vi "DetectDaxsonics.vi"(11 "Main Digitizer":T1=enum."NI Digitizer") -> (1 "Trig Slope":u16(ring) items=["Positive", "Negative"], 2 "Offset Delay (us)":dbl)   [LabVIEW 2022 SP3]
uses:
  Digitizers/-DigitizerRoutines/Digitizer.ctl
  Daxsonics_Pulsers.ctl
  PulserGlobals.vi
panel:
  out "Daxsonics Present":refnum<visa-resource-name>[](array[refnum])
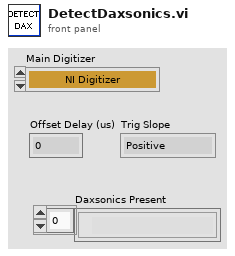
[diagram p1: front panel]
types:
  T1 = typedef "Digitizer.ctl" = enum16{"Acqiris Digitizer", "NI Digitizer", "LeCroy", "GaGe", "AlazarTech", "No Digitizer", "Teledyne"}
  T2 = typedef "Daxsonics_Pulsers.ctl" = enum16{"BP1", "BP2_A", "BP2_B", "10ERS8", "New2021"}
  T3 = enum16{"Left Button", "Center Button", "Right Button", "Window Close"}
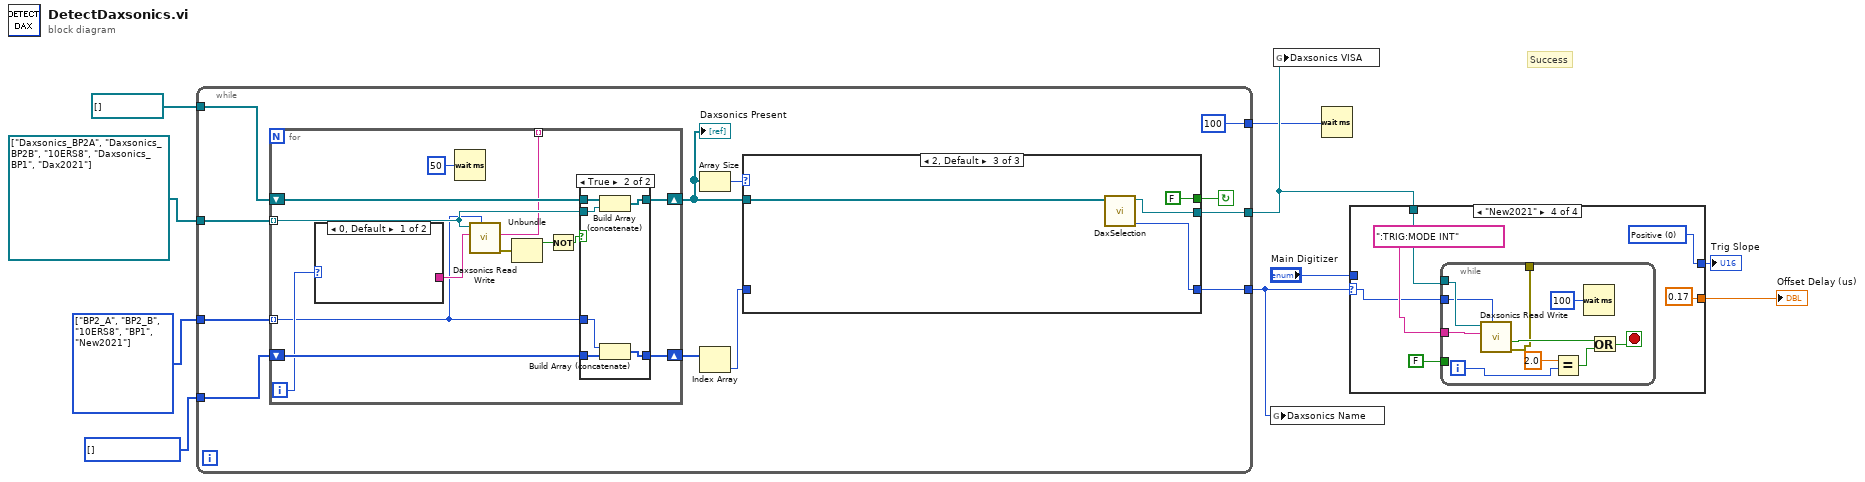
[diagram p0: block diagram]
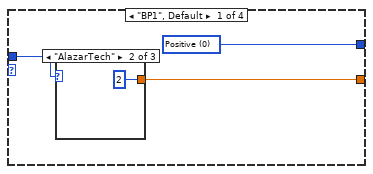
[diagram p2: hidden frame]
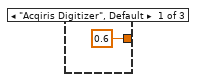
[diagram p3: hidden frame]
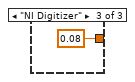
[diagram p4: hidden frame]
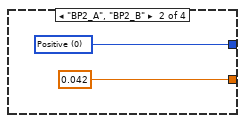
[diagram p5: hidden frame]
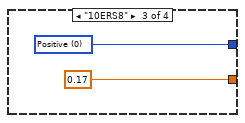
[diagram p6: hidden frame]
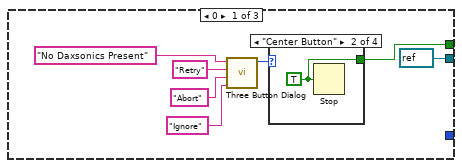
[diagram p7: hidden frame]
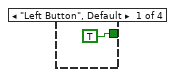
[diagram p8: hidden frame]
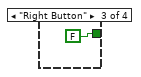
[diagram p9: hidden frame]
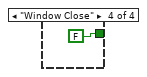
[diagram p10: hidden frame]
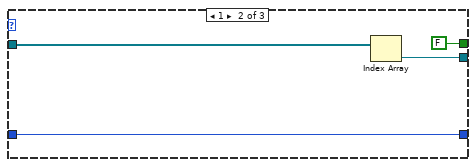
[diagram p11: hidden frame]
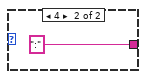
[diagram p12: hidden frame]
diagram:
  w4 = T2[] [] items=["BP1", "BP2_A", "BP2_B", "10ERS8", "New2021"]
  w5 = T2[] [enum."BP2_A", enum."BP2_B", enum."10ERS8", enum."BP1", enum."New2021"] items=["BP1", "BP2_A", "BP2_B", "10ERS8", "New2021"]
  # "Success"
  n1 = while {
    tunnel: [w20] -> w2
    tunnel: [w19] -> w7
    tunnel: refnum<visa-resource-name>[] ["Daxsonics_BP2A", "Daxsonics_BP2B", "10ERS8", "Daxsonics_BP1", "Dax2021"] -> [w15]
    tunnel: w5 -> [w14]
    tunnel: w4 -> [w13]
    tunnel: refnum<visa-resource-name>[] [] -> [w12]
    tunnel: [u32 100 ("milliseconds to wait")] -> w1
    stop <- w16 continue-if-true
    n2 = for {
      tunnel: w15 -> [w50] mode=indexing
      shift-right: [w51] -> w21
      shift-left: w12 -> [w53]
      tunnel: w14 -> [w42] mode=indexing
      shift-right: [w47] -> w17
      shift-left: w13 -> [w48]
      tunnel: [w44] -> _ mode=indexing
      i -> [w46]
      n3 = case shown="0, Default" w46 {
        tunnel: [_ ":"] -> w45
        frame 0, Default {
        }
        frame 4 {
        }
      }
      n4 = Wait (ms)(milliseconds to wait=u32 50) -> ()  [unwired: 1 out]
      n5 = call "Daxsonics Read Write.vi"("Daxsonics Name"=w42, "write buffer"=w45, "VISA resource name"=w50) -> ("error out"=w54:errorcluster, "read buffer"=w44:string)  [unwired: 6 in, 1 out]
      n6 = Unbundle(w54) -> ("status"=w52:bool)  [unwired: 2 out]
      n7 = Not(x=w52) -> (.not. x?=w49:bool)
      n8 = case shown="True" w49 {
        tunnel: [w57 w63] -> w51
        tunnel: w53 -> [w57 w62]
        tunnel: w50 -> [_ w61]
        tunnel: [w56 w60] -> w47
        tunnel: w42 -> [_ w59]
        tunnel: w48 -> [w56 w58]
        frame False {
        }
        frame True {
          n9 = Build Array (concatenate)(w62, w61) -> (w63:refnum<visa-resource-name>[])
          n10 = Build Array (concatenate)(w59, w58) -> (w60:T2[])
        }
      }
    }
    "Daxsonics Present" <- w21
    n11 = Array Size(array=w21) -> (size(s)=w22:i32)
    n12 = Index Array(array=w17) -> (element=w18:T2)  [unwired: 1 in]
    n13 = case shown="2, Default" w22 {
      tunnel: w21 -> [_ w37 w40]
      tunnel: [refnum<visa-resource-name> refnum ("VISA resource name") w36 w41] -> w20
      tunnel: [_ w35 w39] -> w19
      tunnel: w18 -> [_ w35 _]
      tunnel: [w23 FALSE ("T button?") FALSE ("T button?")] -> w16
      frame 0 {
        n14 = call <vilib>:"Three Button Dialog.vi"("Right Button Text (\"Cancel\")"="Ignore" ("Right Button Text (\"Cancel\")"), "Center Button Text (\"No\")"="Abort" ("F button name (\"Cancel\")"), "Left Button Text (\"Yes\")"="Retry" ("T button name (\"OK\")"), "message"="No Daxsonics Present") -> ("Which Button?"=w24:T3)  [unwired: 7 in]
        n15 = case shown="\"Center Button\"" w24 {
          tunnel: [TRUE w31 FALSE FALSE] -> w23
          frame "Left Button", Default {
          }
          frame "Center Button" {
            w31 = TRUE ("stop? (T)")
            n16 = Stop(stop? (T)=w31) -> ()
          }
          frame "Right Button" {
          }
          frame "Window Close" {
          }
        }
      }
      frame 1 {
        n17 = Index Array(array=w37) -> (element=w36:refnum<visa-resource-name>)  [unwired: 1 in]
      }
      frame 2, Default {
        n18 = call "DaxSelection.vi"("Daxsonics Present"=w40) -> ("Daxsonics Name"=w39:T2, "Selected Daxsonics"=w41:refnum<visa-resource-name>)  [unwired: 9 in]
      }
    }
  }
  n19 = global write "PulserGlobals.vi" "Daxsonics Name"(w7) -> ()
  n20 = global write "PulserGlobals.vi" "Daxsonics VISA"(w2) -> ()
  n21 = Wait (ms)(milliseconds to wait=w1) -> ()  [unwired: 1 out]
  n22 = case shown="\"New2021\"" w7 {
    selector: w7 -> [_ _ _ w74]
    tunnel: [w65 0.042 ("Offset delay (us)") 0.17 ("Offset delay (us)") 0.17 ("Offset delay (us)")] -> w9
    tunnel: [w64 w70 w72 w76] -> w8
    tunnel: "Main Digitizer" -> [w66 _ _ _]
    tunnel: w2 -> [_ _ _ w78]
    frame "BP1", Default {
      w64 = u16 0 items=["Positive", "Negative"] ("Trig Slope")
      n23 = case shown="\"AlazarTech\"" w66 {
        tunnel: [0.6 2 0.08] -> w65
        frame "Acqiris Digitizer", Default {
        }
        frame "AlazarTech" {
        }
        frame "NI Digitizer" {
        }
      }
    }
    frame "BP2_A", "BP2_B" {
      w70 = u16 0 items=["Positive", "Negative"] ("Trig Slope")
    }
    frame "10ERS8" {
      w72 = u16 0 items=["Positive", "Negative"] ("Trig Slope")
    }
    frame "New2021" {
      w76 = u16 0 items=["Positive", "Negative"] ("Trig Slope")
      n24 = while {
        tunnel: w78 -> [w89]
        tunnel: ":TRIG:MODE INT" -> [w88]
        tunnel: FALSE ("CR on Write?") -> [_]
        tunnel: [w81] -> _
        tunnel: w74 -> [w80]
        i -> [w86]
        stop <- w84 stop-if-true
        n25 = call "Daxsonics Read Write.vi"("Daxsonics Name"=w80, "write buffer"=w88, "VISA resource name"=w89) -> ("error out"=w81:errorcluster, "Success?"=w83:bool)  [unwired: 6 in, 1 out]
        n26 = Equal?(x=2.0, y=w86) -> (x = y?=w85:bool)
        n27 = Wait (ms)(milliseconds to wait=u32 100) -> ()  [unwired: 1 out]
        n28 = Or(x=w83, y=w85) -> (x .or. y?=w84:bool)
      }
    }
  }
  "Offset Delay (us)" <- w9
  "Trig Slope" <- w8
